vi "Analysator Seriennummer und Type ermitteln.vi"(7 "byName":bool, 11 "Analysator":T1) -> (1 "Seriennummer":string, 2 "Type":string, 3 "Name für Protokoll":string)   [LabVIEW 2020, in "System Einstellungen V2.lvlib"]
uses:
  System Einstellungen V2.lvlib
  Analysatoren.ctl
  Aktion FGV SystemEinstellungenV2.ctl
  AnalysatorDefinition.ctl
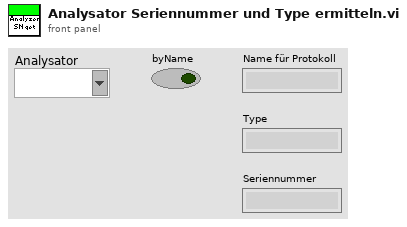
[diagram p1: front panel]
types:
  T1 = typedef "System Einstellungen V2.lvlib/Analysatoren.ctl" = string
  T2 = typedef "System Einstellungen V2.lvlib/AnalysatorDefinition.ctl" = cluster{"Analysator":string, "Name für Protokoll":string, "Type":string, "Seriennummer":string}
  T3 = typedef "System Einstellungen V2.lvlib/Aktion FGV SystemEinstellungenV2.ctl" = enum16{"lesen", "Analysatoren schreiben", "Analysator ändern", "Analysatoren löschen", "laden", "speichern", "Untertitel", "Analysatoren", "Neue Analysatoren", "Gasteiler schreiben", "Gasteiler ändern", "Gasteiler löschen", "Gasteiler", "Gasteiler exportieren", "Gasteiler importieren"}
  T4 = typedef "LVComboBoxStrsAndValuesArrayTypeDef.ctl" = cluster{"String":string, "Value":string}[]
  T5 = cluster{"AnalysatorDefinitionListe":T2[], "AnalysatorDefinitionTextListe":string[][], "Analysatoren Strings And Values[]":T4}
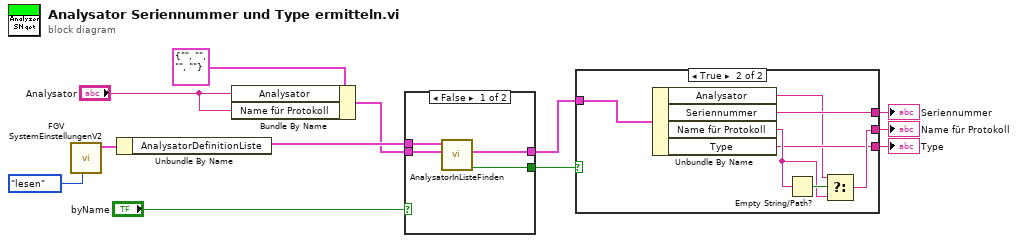
[diagram p0: block diagram]
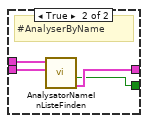
[diagram p2: hidden frame]
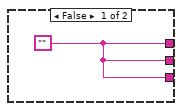
[diagram p3: hidden frame]
diagram:
  n1 = call "FGV SystemEinstellungenV2.vi"("Aktion"=Aktion_FGV_SystemEinstellungenV2."lesen") -> ("Analysatoren"=w10:T5)  [unwired: 5 in, 5 out]
  n2 = Unbundle By Name(w10) -> ("AnalysatorDefinitionListe"=w6:T2[])
  n3 = Bundle By Name(cluster=T2 {"Analysator"="", "Name für Protokoll"="", "Type"="", "Seriennummer"=""} ("AnalysatorDefinition"), "Analysator"="Analysator", "Name für Protokoll"="Analysator") -> (w4:T2)
  n4 = case shown="False" "byName" {
    tunnel: w6 -> [w15 w20]
    tunnel: w4 -> [w16 w19]
    tunnel: [w14 w18] -> w3
    tunnel: [w13 w17] -> w2
    frame False {
      n5 = call "AnalysatorInListeFinden.vi"("AnalysatorDefinition"=w16, "AnalysatorListe"=w15) -> ("gefunden"=w13:bool, "AnalysatorDefinition out"=w14:T2)  [unwired: 6 in, 2 out]
    }
    frame True {
      # "#AnalyserByName"
      n6 = call "AnalysatorNameInListeFinden.vi"("AnalysatorDefinition"=w19, "AnalysatorListe"=w20) -> ("Analysator"=w18:T2, "gefunden"=w17:bool)  [unwired: 6 in, 2 out]
    }
  }
  n7 = case shown="True" w2 {
    tunnel: w3 -> [_ w23]
    tunnel: [w21 w28] -> w12
    tunnel: [w21 w25] -> w9
    tunnel: [w21 w24] -> w8
    frame False {
      w21 = ""
    }
    frame True {
      n8 = Unbundle By Name(w23) -> ("Analysator"=w22:string, "Seriennummer"=w28:string, "Name für Protokoll"=w26:string, "Type"=w24:string)
      n9 = Empty String/Path?(string/path=w26) -> (empty?=w27:bool)
      n10 = Select(t=w22, s=w27, f=w26) -> (s? t:f=w25:string)
    }
  }
  "Seriennummer" <- w12
  "Name für Protokoll" <- w9
  "Type" <- w8
